vi "stop_write.vi"(7 "references":T1, 8 "error in (no error)":errorcluster, 11 "stop":bool=TRUE) -> (0 "error out":errorcluster)   [LabVIEW 2015, in "lv-recipe-machine.lvlib"]
doc: "This VI can be used to set or unset the internal stop notifier privately. Generally it's called only once when the module receives the die command via the input_queue."
uses:
  lv-recipe-machine.lvlib
  public/_controls/references.ctl
  public/_controls/input.ctl
  public/_controls/input_command.ctl
  public/_controls/output.ctl
  public/_controls/data.ctl
  public/_controls/configuration.ctl
  public/_controls/recipe_data.ctl
  public/_controls/mode.ctl
  public/_controls/manual_state.ctl
  public/_controls/automatic_state.ctl
  public/_controls/recipe_step.ctl
  <userlib>/antonio-alexander/lv-waitgroup/public/_controls/api_waitgroup.ctl
  public/_controls/change.ctl
  public/_controls/status.ctl
  <userlib>/antonio-alexander/lv-waitgroup/lv-waitgroup.lvlib
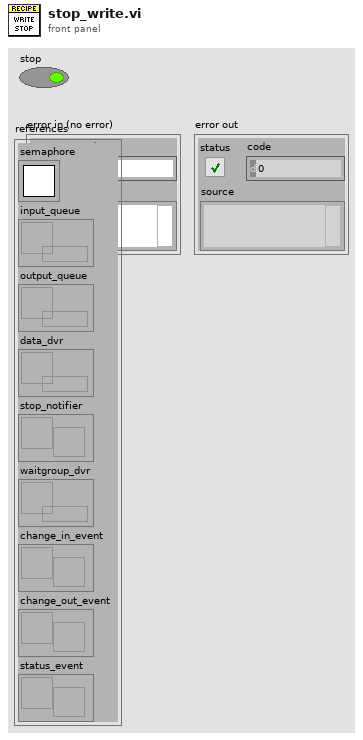
[diagram p1: front panel]
types:
  T1 = typedef "lv-recipe-machine.lvlib/references.ctl" = cluster{"semaphore":T2, "input_queue":refnum<queue>, "output_queue":refnum<queue>, "data_dvr":refnum<data-value>, "stop_notifier":refnum<notifier>, "waitgroup_dvr":refnum<data-value>, "change_in_event":refnum<user-event>, "change_out_event":refnum<user-event>, "status_event":refnum<user-event>}
  T2 = typedef "Semaphore RefNum" = refnum<k1>
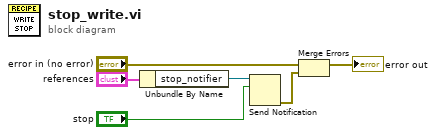
[diagram p0: block diagram]
diagram:
  n1 = Unbundle By Name("references") -> ("stop_notifier"=w4:refnum<notifier>)
  n2 = Send Notification(notification="stop", notifier=w4) -> (error out=w6:errorcluster)  [unwired: 1 in, 1 out]
  n3 = Merge Errors("error in (no error)", w6) -> (→"error out":errorcluster)
